vi "UHR-Fleezers Control (host) -TL FB Corrected Ronen.vi"(0 "Tab Control":T5(tab)=enum."DAQ AI") -> ()   [LabVIEW 2013] (continued)
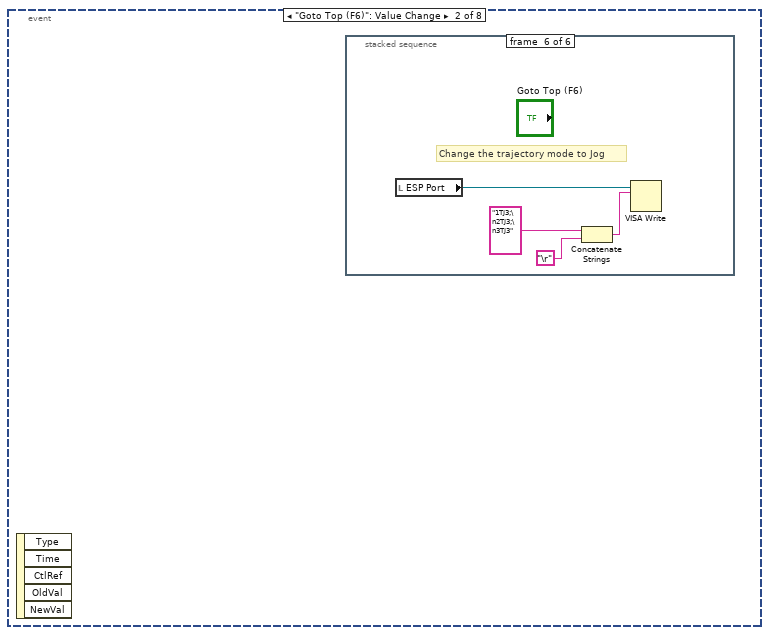
[diagram p4: hidden frame]
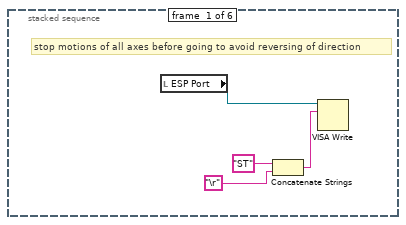
[diagram p5: hidden frame]
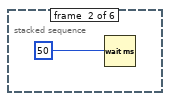
[diagram p6: hidden frame]
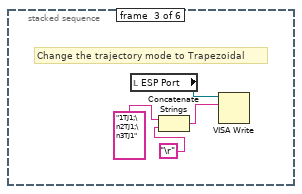
[diagram p7: hidden frame]
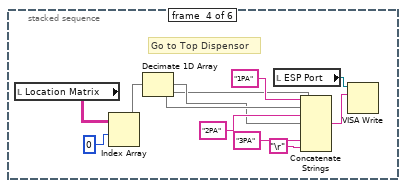
[diagram p8: hidden frame]
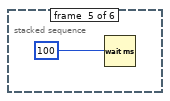
[diagram p9: hidden frame]
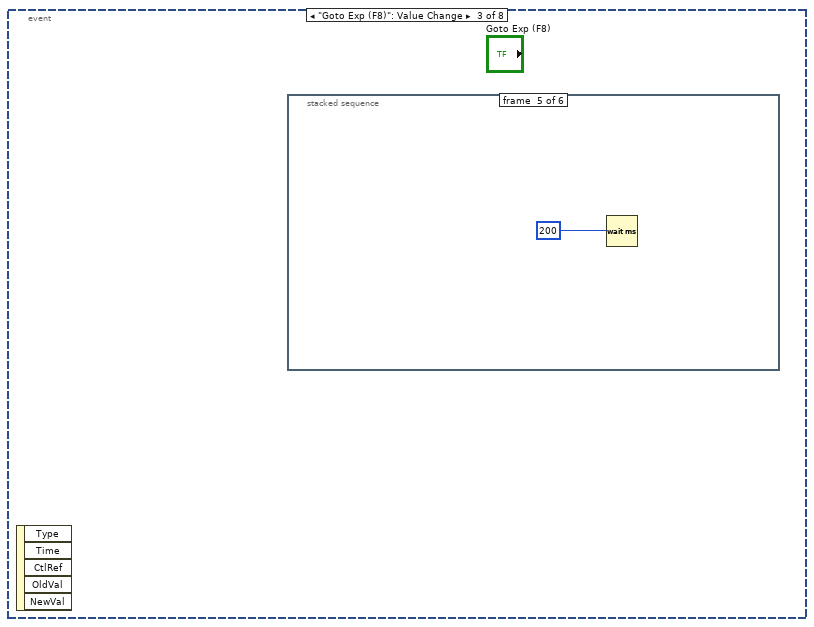
[diagram p10: hidden frame]
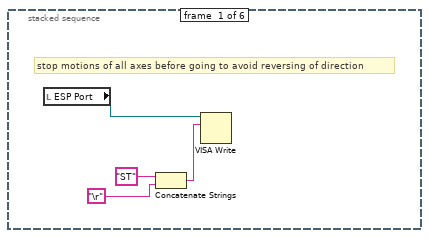
[diagram p11: hidden frame]
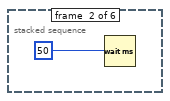
[diagram p12: hidden frame]
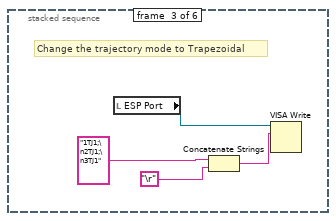
[diagram p13: hidden frame]
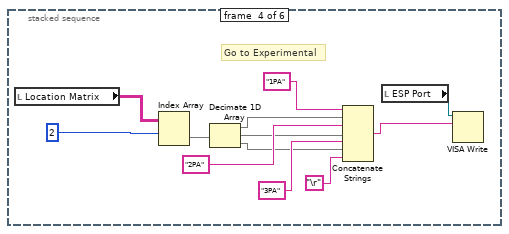
[diagram p14: hidden frame]
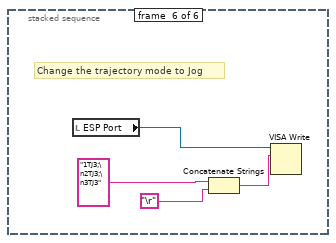
[diagram p15: hidden frame]
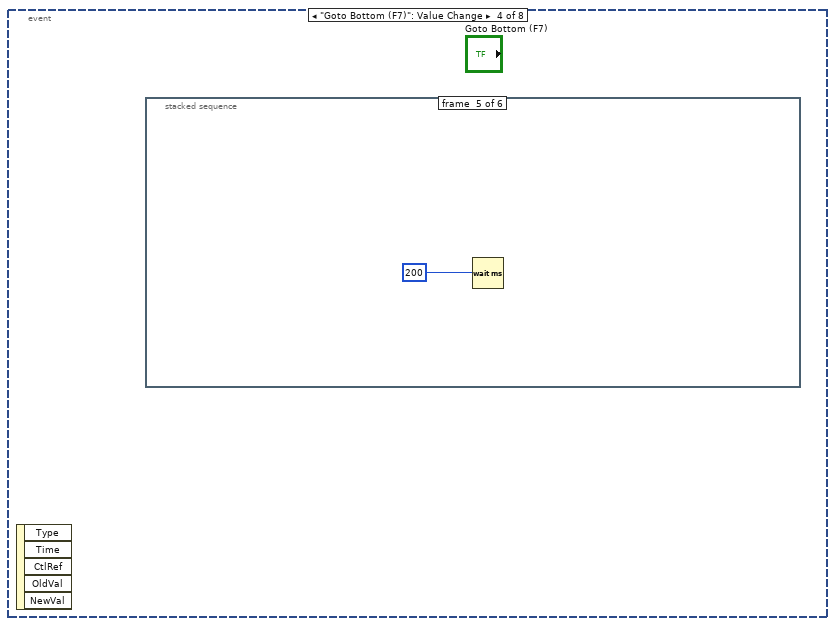
[diagram p16: hidden frame]
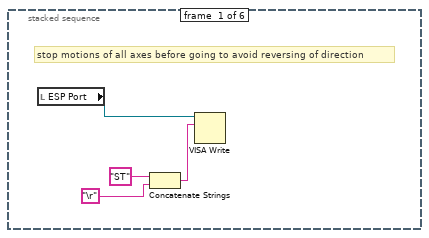
[diagram p17: hidden frame]
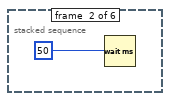
[diagram p18: hidden frame]
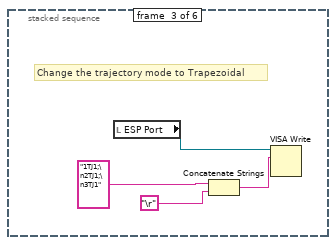
[diagram p19: hidden frame]
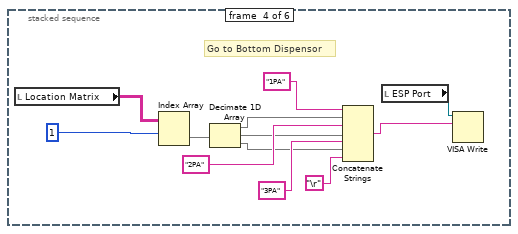
[diagram p20: hidden frame]
                          n2310 = local write "Fish for Tether"(FALSE ("Fish for Tether")) -> ()
                          n2311 = call <vilib>:"Beep.vi"() -> ()  [unwired: 3 in, 9 out]
                          n2312 = local read "Messages"() -> (w3850:string)
                          n2313 = call "Update messages.vi"("Message to add"="Tether fishing timeout." ("Messages"), "Old message string"=w3850) -> ("New message string"=→"Messages":string)
                        }
                      }
                    }
                  }
                  n2314 = local read "Y RF Frequency Limits (MHz)"() -> (w3809:T17)
                  n2315 = local read "X RF Frequency Limits (MHz)"() -> (w3810:T17)
                  n2316 = local read "BD 1 Frequency 3 (MHz)"() -> (w3815:dbl)
                  n2317 = local read "BD 2 Frequency 2 (MHz)"() -> (w3799:dbl)
                  n2318 = Select(t=w3800, s="Scan axis 2", f=w3799) -> (s? t:f=w3811:dbl)
                  n2319 = Add(x=w3808, y=w3811) -> (x+y=w3806:dbl)
                  n2320 = Select(t=w3806, s="Scan axis 2", f=w3800) -> (s? t:f=w3798:dbl)
                  n2321 = Select(t=w3799, s="Scan axis 2", f=w3806) -> (s? t:f=w3813:dbl)
                  n2322 = local read "BD 2 Frequency 3 (MHz)"() -> (w3814:dbl)
                  n2323 = call "set RF board frequency - interlace.vi"("Board 2 Frequency Limits"=w3809, "Board 1 Frequency Limits"=w3810, "FPGA VI Reference In"=w3805, "Board 2 Frequency 3 (MHz)"=w3814, "Board 1 Frequency 3 (MHz)"=w3815, "Board 2 Frequency 2 (MHz)"=w3799, "Board 2 Frequency 1 (MHz)"=w3813, "Board 1 Frequency 2 (MHz)"=w3798, "Board 1 Frequency 1  (MHz)"=w3797) -> ()  [unwired: 1 in, 2 out]
                }
                frame #1 {
                  n2324 = And(x=w3858, y=w3855) -> (x .and. y?=w3857:bool)
                  n2325 = case "Only if were fishing and now formed tether" shown="True" w3857 {
                    tunnel: w3856 -> [w3860 w3872]
                    tunnel: [w3859 w3871] -> w3854
                    tunnel: w3853 -> [_ w3867]
                    frame False {
                      n2326 = local read "Fish for Tether"() -> (w3859:bool)
                      n2327 = case shown="True" w3859 {
                        tunnel: w3860 -> [_ _]
                        frame False {
                        }
                        frame True {
                        }
                      }
                    }
                    frame True {
                      w3871 = FALSE ("Fish for Tether")
                      n2328 = call <vilib>:"Beep.vi"() -> ()  [unwired: 3 in, 9 out]
                      n2329 = Number To Decimal String(number=w3867, width (-)=i16 1) -> (decimal integer string=w3865:string)
                      n2330 = case shown="\"2\", \"3\", \"4\", \"5\", \"6\"" "Then..." {
                        selector: "Then..." -> [_ w3875]
                        tunnel: w3872 -> [w3874 _]
                        frame "1", Default {
                          # "do nothing"
                          n2331 = property on="BD 1 Frequency 1 (MHz)" class="DigNum (strict)"("Val(Sgnl)"=w3874) -> ()  [unwired: 2 in, 2 out]
                        }
                        frame "2", "3", "4", "5", "6" {
                          n2332 = flat-sequence {
                            tunnel: w3875 -> [w3877]
                            frame #0 {
                              n2333 = property on="Trap Delta (MHz)" class="DigNum (strict)"("Val(Sgnl)"="Move to Delta 1 (MHz)") -> ()  [unwired: 2 in, 2 out]
                            }
                            frame #1 {
                              n2334 = case shown="\"5\", \"6\"" w3877 {
                                selector: w3877 -> [w3880 w3890 _]
                                frame "3", "4" {
                                n2335 = flat-sequence {
                                tunnel: w3880 -> [w3881]
                                tunnel: [w3881] -> w3878
                                tunnel: [w3883] -> w3879
                                tunnel: w3878 -> [w3883]
                                tunnel: w3879 -> [w3887]
                                frame #0 {
                                n2336 = property on="Green Laser ON/Interlacing" class="Bool (strict)"("Val(Sgnl)"=TRUE ("Value (Signaling)")) -> ()  [unwired: 2 in, 2 out]
                                }
                                frame #1 {
                                n2337 = Multiply(x="Wait Before Save (s)", y=u32 1000 ("x")) -> (x*y=w3885:u32)
                                n2338 = Wait (ms)(milliseconds to wait=w3885) -> ()  [unwired: 1 out]
                                }
                                frame #2 {
                                n2339 = property on="Start Saving" class="Bool (strict)"("Value"=TRUE ("Start Saving")) -> ()  [unwired: 2 in, 2 out]
                                n2340 = case shown="Default" w3887 {
                                frame Default {
                                }
                                frame "4" {
                                n2341 = property on="Fl. Triggered..." class="Bool (strict)"("Val(Sgnl)"=TRUE ("Value (Signaling)")) -> ()  [unwired: 2 in, 2 out]
                                }
                                }
                                }
                                }
                                }
                                frame "5", "6" {
                                n2342 = stacked-sequence {
                                tunnel: w3890 -> [_ _ _ _ _ _ _ _ w3907 _ _]
                                frame #0 {
                                n2343 = Replace Array Subset(array=u32[] [0] ("Index Values"), new element="Raster Set Upon Tether", index=0) -> (w3891:u32[])
                                n2344 = property on="Saved AOD Raster Scan Parameter Sets" class="Arr (strict)"("Index Values"=w3891) -> ()  [unwired: 2 in, 2 out]
                                }
                                frame #1 {
                                n2345 = Wait (ms)(milliseconds to wait=u32 500) -> ()  [unwired: 1 out]
                                }
                                frame #2 {
                                n2346 = property on="Load parameters" class="Bool (strict)"("Val(Sgnl)"=TRUE ("Value (Signaling)")) -> ()  [unwired: 2 in, 2 out]
                                }
                                frame #3 {
                                n2347 = Wait (ms)(milliseconds to wait=u32 500) -> ()  [unwired: 1 out]
                                }
                                frame #4 {
                                n2348 = property on="Trap Raster Scan" class="Bool (strict)"("Val(Sgnl)"=TRUE ("Value (Signaling)")) -> ()  [unwired: 2 in, 2 out]
                                }
                                frame #5 {
                                n2349 = Wait (ms)(milliseconds to wait=u32 2000) -> ()  [unwired: 1 out]
                                }
                                frame #6 {
                                n2350 = while {
                                stop <- w3902 stop-if-true
                                n2351 = local read "Raster Scanning..."() -> (w3901:bool)
                                n2352 = local read "Saving..."() -> (w3904:bool)
                                n2353 = Wait (ms)(milliseconds to wait=u32 100) -> ()  [unwired: 1 out]
                                n2354 = Not(x=w3904) -> (.not. x?=w3903:bool)
                                n2355 = Not(x=w3901) -> (.not. x?=w3900:bool)
                                n2356 = And(x=w3903, y=w3900) -> (x .and. y?=w3902:bool)
                                }
                                }
                                frame #7 {
                                n2357 = property on="Trap Delta (MHz)" class="DigNum (strict)"("Val(Sgnl)"="Move to Delta 2 (MHz)") -> ()  [unwired: 2 in, 2 out]
                                }
                                frame #8 {
                                n2358 = local read "Tether"() -> (w3908:bool)
                                n2359 = case shown="True" w3908 {
                                tunnel: w3907 -> [_ w3909]
                                frame False {
                                }
                                frame True {
                                n2360 = flat-sequence {
                                tunnel: w3909 -> [w3911]
                                frame #0 {
                                n2361 = Wait (ms)(milliseconds to wait=u32 500) -> ()  [unwired: 1 out]
                                }
                                frame #1 {
                                n2362 = case shown="\"6\"" w3911 {
                                frame Default {
                                }
                                frame "6" {
                                n2363 = property on="Green Laser ON/Interlacing" class="Bool (strict)"("Val(Sgnl)"=TRUE ("Green Laser ON/Interlacing")) -> ()  [unwired: 2 in, 2 out]
                                }
                                }
                                }
                                frame #2 {
                                n2364 = Wait (ms)(milliseconds to wait=u32 500) -> ()  [unwired: 1 out]
                                }
                                frame #3 {
                                n2365 = local write "Start Saving"("Save at end (5, 6)") -> ()
                                }
                                }
                                }
                                }
                                }
                                frame #9 {
                                n2366 = local read "Bead Sep. Int. Time (s)"() -> (w3917:dbl)
                                n2367 = Multiply(x=w3917, y=1000.0) -> (x*y=w3916:dbl)
                                n2368 = Wait (ms)(milliseconds to wait=w3916) -> ()  [unwired: 1 out]
                                }
                                frame #10 {
                                n2369 = property on="Rescale on Mean" class="Bool (strict)"("Val(Sgnl)"=TRUE ("Value (Signaling)")) -> ()  [unwired: 2 in, 2 out]
                                }
                                }
                                }
                                frame "2", Default {
                                }
                              }
                            }
                          }
                        }
                      }
                      n2370 = Concatenate Strings("Formed tether in ", w3865, " attempt(s)." ("string")) -> (w3862:string)
                      n2371 = local read "Messages"() -> (w3869:string)
                      n2372 = local write "Fish for Tether"(w3871) -> ()
                      n2373 = call "Update messages.vi"("Message to add"=w3862, "Old message string"=w3869) -> ("New message string"=w3868:string)
                      n2374 = local write "Messages"(w3868) -> ()
                      n2375 = Get Date/Time In Seconds() -> (seconds since 1Jan1904=→"Time tether formed":timestamp)
                      "Tether" <- "Tether Alarm?"
                    }
                  }
                }
                frame #2 {
                  n2376 = local read "Oscillate Set 2"() -> (w3921:bool)
                  n2377 = local read "Stop All"() -> (w3923:bool)
                  n2378 = Not Or(1:w3920, 2:w3921) -> (0:w3919:bool)
                  n2379 = Compound Arithmetic op=OR(w3923, w3919) -> (w3922:bool)
                }
              }
              n2380 = node-c288() -> ()  [unwired: 2 out]
            }
            n2381 = node-c288(w3783) -> ()  [unwired: 1 out]
          }
        }
      }
      event "Fl. Triggered...": Value Change {
        n2382 = event-data() -> ()  [unwired: 7 out]
        n2383 = case shown="True" "Fl. Triggered..." {
          frame False {
          }
          frame True {
            n2384 = node-c288() -> (w3935:T25)  [unwired: 4 out]
            n2385 = timed-loop {
              timing: w3935 -> [_]
              timing-out: [_] -> w3934
              tunnel: "Action" -> [w3939]
              shift-right: [w3936] -> _
              shift-left: u8 255 -> [w3938]
              stop <- w3940 stop-if-true
              n2386 = node-c288() -> ()  [unwired: 2 out]
              n2387 = flat-sequence {
                tunnel: w3939 -> [w3952]
                tunnel: w3938 -> [w3949]
                tunnel: [w3948] -> w3937
                tunnel: [w4038] -> w3940
                tunnel: w3937 -> [w4037]
                tunnel: [w4037] -> w3936
                frame #0 {
                  n2388 = local read "Delta Fl. 2"() -> (w3943:dbl)
                  n2389 = local read "Delta Fl. 1"() -> (w3944:dbl)
                  n2390 = Select(t=w3944, s="APD to Watch", f=w3943) -> (s? t:f=w3942:dbl)
                  n2391 = Multiply(x="Fl. Delta Thresh. (kHz)", y=1000.0) -> (x*y=w3951:dbl)
                  n2392 = Greater?(x=w3942, y=w3951) -> (0:w3946:bool)
                  n2393 = Or(x="Force Yank", y=w3946) -> (x .or. y?=w3947:bool)
                  n2394 = case shown="True" w3947 {
                    tunnel: w3952 -> [_ w3962]
                    tunnel: w3949 -> [w3954 w3958]
                    tunnel: [w3954 w3955] -> w3948
                    frame False {
                    }
                    frame True {
                      n2395 = flat-sequence {
                        tunnel: w3959 -> [w3968]
                        tunnel: [w3968] -> w3963
                        tunnel: w3962 -> [w3967]
                        tunnel: [w3967] -> w3961
                        tunnel: [w3966] -> w3960
                        tunnel: w3958 -> [w3965]
                        tunnel: [w3964] -> w3957
                        tunnel: w3963 -> [w3993]
                        tunnel: w3961 -> [w3992]
                        tunnel: w3960 -> [w3991]
                        tunnel: w3957 -> [w3990]
                        tunnel: [w3990] -> w3956
                        tunnel: w3956 -> [w4035]
                        tunnel: [w4035] -> w3955
                        frame #0 {
                          n2396 = call <vilib>:"Beep.vi"() -> ()  [unwired: 3 in, 9 out]
                          n2397 = local write "Waiting"(FALSE ("Waiting")) -> ()
                          n2398 = Increment(x=w3965) -> (x+1=w3964:u8)
                          n2399 = case shown="\"Yank\"" w3967 {
                            tunnel: w3964 -> [_ _ w3974]
                            frame "Image" {
                              n2400 = property on="Confocal Image" class="Bool (strict)"("Val(Sgnl)"=TRUE ("Value (Signaling)")) -> ()  [unwired: 2 in, 2 out]
                            }
                            frame "Alarm", Default {
                            }
                            frame "Yank" {
                              n2401 = flat-sequence {
                                tunnel: w3974 -> [w3977]
                                tunnel: [w3976] -> w3973
                                tunnel: ["N Array El"] -> w3972
                                tunnel: w3973 -> [w3987]
                                tunnel: w3972 -> [w3983]
                                frame #0 {
                                n2402 = Multiply(x="Yank Delay (s)", y=1000.0) -> (x*y=w3980:dbl)
                                n2403 = Quotient & Remainder(x=w3977, y="N Array El") -> (x-y*floor(x/y)=w3976:u8)  [unwired: 1 out]
                                n2404 = Wait (ms)(milliseconds to wait=w3980) -> ()  [unwired: 1 out]
                                }
                                frame #1 {
                                n2405 = Random Number (0-1)() -> (number: 0 to 1=w3984:dbl)
                                n2406 = Multiply(x=w3983, y=w3984) -> (x*y=w3982:dbl)
                                n2407 = Round Toward -Infinity(1:w3982) -> (0:w3981:dbl)
                                n2408 = Select(t=w3981, s="Random Choice", f=w3987) -> (s? t:f=w3985:dbl)
                                n2409 = Index Array(array="Yank to Delta Array (MHz)", index=w3985) -> (element=w3988:dbl)
                                n2410 = property on="Trap Delta (MHz)" class="DigNum (strict)"("Val(Sgnl)"=w3988) -> ()  [unwired: 2 in, 2 out]
                                }
                              }
                            }
                          }
                          n2411 = local read "Time (s)"() -> (w3966:dbl)
                          "Fl. High" <- TRUE ("Yanking")
                        }
                        frame #1 {
                          n2412 = node-c288() -> (w3995:T25)  [unwired: 4 out]
                          n2413 = timed-loop {
                            timing: w3995 -> [_]
                            timing-out: [_] -> w3994
                            tunnel: w3993 -> [w4011]
                            tunnel: w3992 -> [w4009]
                            tunnel: w3991 -> [w4008]
                            stop <- w4010 stop-if-true
                            n2414 = node-c288() -> ()  [unwired: 2 out]
                            n2415 = local read "Fl. Delta Thresh. (kHz)"() -> (w4003:dbl)
                            n2416 = local read "Fl. Triggered..."() -> (w4012:bool)
                            n2417 = local read "Delta Fl. 1"() -> (w3999:dbl)
                            n2418 = local read "Delta Fl. 2"() -> (w3997:dbl)
                            n2419 = local read "Stop All"() -> (w4006:bool)
                            n2420 = local read "APD to Watch"() -> (w3998:bool)
                            n2421 = Select(t=w3999, s=w3998, f=w3997) -> (s? t:f=w3996:dbl)
                            n2422 = Not(x=w4012) -> (.not. x?=w4007:bool)
                            n2423 = Multiply(x=w4003, y=1000.0) -> (x*y=w4002:dbl)
                            n2424 = Negate(x=w4002) -> (-x=w4001:dbl)
                            n2425 = Less?(x=w3996, y=w4001) -> (x < y?=w4005:bool)
                            n2426 = Compound Arithmetic op=OR(w4005, w4006, w4007, "Force Reset") -> (w4010:bool)
                            n2427 = case shown="True" w4010 {
                              tunnel: w4011 -> [_ w4023]
                              tunnel: w4009 -> [_ w4022]
                              tunnel: w4008 -> [_ w4020]
                              frame False {
                              }
                              frame True {
                                n2428 = case shown="\"Yank\"" w4022 {
                                tunnel: w4023 -> [_ w4024]
                                frame "Image", Default {
                                }
                                frame "Yank" {
                                n2429 = flat-sequence {
                                tunnel: [w4029] -> w4025
                                tunnel: w4024 -> [w4029]
                                tunnel: w4025 -> [w4030]
                                frame #0 {
                                n2430 = local read "Yank Delay (s)"() -> (w4028:dbl)
                                n2431 = Multiply(x=w4028, y=1000.0) -> (x*y=w4026:dbl)
                                n2432 = Wait (ms)(milliseconds to wait=w4026) -> ()  [unwired: 1 out]
                                }
                                frame #1 {
                                n2433 = property on="Trap Delta (MHz)" class="DigNum (strict)"("Val(Sgnl)"=w4030) -> ()  [unwired: 2 in, 2 out]
                                }
                                }
                                }
                                }
                                n2434 = local read "Time (s)"() -> (w4021:dbl)
                                n2435 = Subtract(x=w4021, y=w4020) -> (x-y=w4017:dbl)
                                "Duration (s)" <- w4017
                                n2436 = Number To Decimal String(number=w4017, width (-)=i16 0) -> (decimal integer string=w4015:string)
                                n2437 = Concatenate Strings(w4015, " s fluorescence event." ("string")) -> (w4013:string)
                                n2438 = local read "Messages"() -> (w4019:string)
                                n2439 = call "Update messages.vi"("Message to add"=w4013, "Old message string"=w4019) -> ("New message string"=w4018:string)
                                n2440 = call <vilib>:"Beep.vi"() -> ()  [unwired: 3 in, 9 out]
                                n2441 = local write "Messages"(w4018) -> ()
                              }
                            }
                            n2442 = node-c288() -> ()  [unwired: 2 out]
                          }
                          n2443 = node-c288(w3994) -> ()  [unwired: 1 out]
                        }
                        frame #2 {
                          n2444 = local write "Fl. High"(FALSE ("Yanking")) -> ()
                        }
                      }
                      n2445 = local read "Trap Delta (MHz)"() -> (w3959:dbl)
                    }
                  }
                }
                frame #1 {
                  n2446 = local read "Stop All"() -> (w4041:bool)
                  n2447 = local read "Fl. Triggered..."() -> (w4039:bool)
                  n2448 = Not(x=w4039) -> (.not. x?=w4040:bool)
                  n2449 = Or(x=w4040, y=w4041) -> (x .or. y?=w4038:bool)
                  n2450 = Not(x=w4038) -> (.not. x?=→"Waiting":bool)
                }
              }
              n2451 = node-c288() -> ()  [unwired: 2 out]
            }
            n2452 = node-c288(w3934) -> ()  [unwired: 1 out]
          }
        }
      }
      event "Stop All": Value Change {
        n2453 = event-data() -> ()  [unwired: 7 out]
        n2454 = local read "Stop All"() -> (w4047:bool)
      }
    }
    n2455 = node-c288() -> ()  [unwired: 2 out]
  }
  n2456 = node-c288(w93) -> ()  [unwired: 1 out]
  n2457 = node-c288(w181) -> ()  [unwired: 1 out]
  n2458 = flat-sequence {
    tunnel: w53 -> [w4052]
    tunnel: [w4051] -> w59
    tunnel: [w4048] -> w58
    tunnel: w57 -> [_]
    tunnel: w56 -> [_]
    tunnel: w55 -> [_]
    tunnel: w54 -> [_]
    tunnel: w52 -> [w4049]
    tunnel: w59 -> [w4055]
    tunnel: w58 -> [w4054]
    frame #0 {
      w4050 = FALSE ("APD to FIFO")
      n2459 = xnode "Read/Write Control"("FPGA VI Reference In"=w4052, "error in"=w4049, "APD to FIFO"=w4050, "AI to FIFO"=w4050) -> ("FPGA VI Reference Out"=w4051:T20, "error out"=w4048:errorcluster)
    }
    frame #1 {
      n2460 = xnode "Invoke Method"("FPGA VI Reference In"=w4055, "error in"=w4054) -> ("FPGA VI Reference Out"=w4053:T20)  [unwired: 1 out]
      n2461 = xnode "Close FPGA VI Reference"("FPGA VI Reference In"=w4053) -> ()  [unwired: 1 in, 1 out]
    }
  }
